vi "Edit Key Dialog.vi"(8 "error in":errorcluster, 10 "Key Name":string, 11 "Config in":refnum<class "Config.lvclass">) -> (0 "error out":errorcluster, 3 "Config out":refnum<class "Config.lvclass">)   [LabVIEW 2023, in "Config.lvlib" / "Config.lvclass"]
uses:
  Config.lvclass
panel:
  out "Dialog":string
  in  "Cancel Button":bool
  in  "OK Button":bool
  in  "Key Value":string
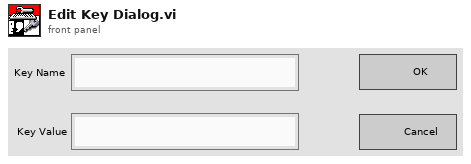
[diagram p1: front panel]
types:
  T1 = enum8{"Enabled", "Disabled", "Disabled and Grayed Out"}
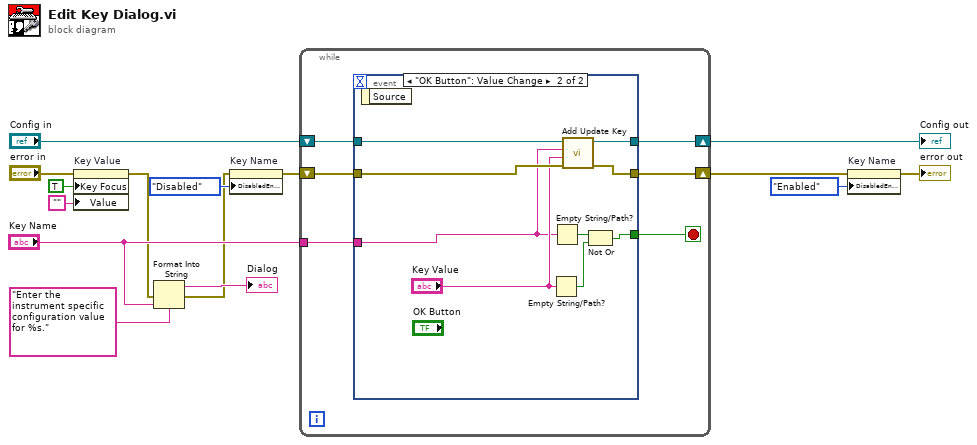
[diagram p0: block diagram]
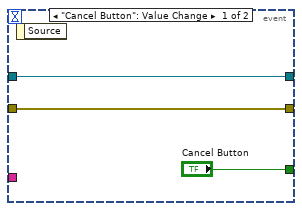
[diagram p2: hidden frame]
diagram:
  n1 = property on="Key Value" class="Str"(error in="error in", "Key Focus"=TRUE, "Value"="") -> (error out=w4:errorcluster)  [unwired: 1 in, 1 out]
  n2 = Format Into String(format string="Enter the instrument specific configuration value for %s.", error in=w4, "Key Name") -> (resulting string=→"Dialog":string, error out=w1:errorcluster)  [unwired: 1 in]
  n3 = property on="Key Name" class="Str"(error in=w1, "DisabledEnum"=T1."Disabled" ("Disabled")) -> (error out=w3:errorcluster)  [unwired: 1 in, 1 out]
  n4 = while {
    shift-right: [w20] -> w14
    shift-left: "Config in" -> [w21]
    shift-right: [w19] -> w7
    shift-left: w3 -> [w18]
    tunnel: "Key Name" -> [w16]
    stop <- w17 stop-if-true
    n5 = event shown="[1] \"OK Button\": Value Change" {
      selector: _ -> [_ _]
      dyn-events: _ -> [_ _]
      timeout: _ -> [_ _]
      tunnel: w21 -> [w24 w32]
      tunnel: [w24 w33] -> w20
      tunnel: [w23 w31] -> w19
      tunnel: w18 -> [w23 w30]
      tunnel: ["Cancel Button" w26] -> w17
      tunnel: w16 -> [_ w25]
      event "Cancel Button": Value Change {
        n6 = event-data() -> ()  [unwired: 1 in, 1 out]
      }
      event "OK Button": Value Change {
        n7 = event-data() -> ()  [unwired: 1 in, 1 out]
        n8 = Empty String/Path?(string/path="Key Value") -> (empty?=w28:bool)
        n9 = Empty String/Path?(string/path=w25) -> (empty?=w27:bool)
        n10 = call "Add Update Key.vi"("error in"=w30, "Value"="Key Value", "Key"=w25, "Config in"=w32) -> ("error out"=w31:errorcluster, "Config out"=w33:refnum<class "Config.lvclass">)  [unwired: 6 in]
        n11 = Not Or(1:w28, 2:w27) -> (0:w26:bool)
      }
    }
  }
  "Config out" <- w14
  n12 = property on="Key Name" class="Str"(error in=w7, "DisabledEnum"=T1."Enabled" ("Disabled")) -> (error out=→"error out":errorcluster)  [unwired: 1 in, 1 out]
